vi "Get Calibration Info.vi"(4 "출장교정 List":refnum<vi>, 5 "교정환경 in":T1, 6 "교정절차 목록 List":refnum<vi>, 7 "교정정보 in":T2 caption="입력 클러스터", 8 "에러 입력(에러 없음)":errorcluster, 9 "콤보박스 참조":refnum<vi>[](array[refnum]), 10 "현장리스트?":bool, 11 "등록번호":string) -> (0 "에러 출력":errorcluster, 1 "교정환경 out":T1, 2 "교정정보 out":T2 caption="출력 클러스터", 3 "기타정보":string[](array[string]))   [LabVIEW 2020]
uses:
  Controls/Clst_Cal Info Global.ctl
  Controls/Clst_Atm Info Global.ctl
  <vilib>/addons/database/NI_Database_API.lvlib
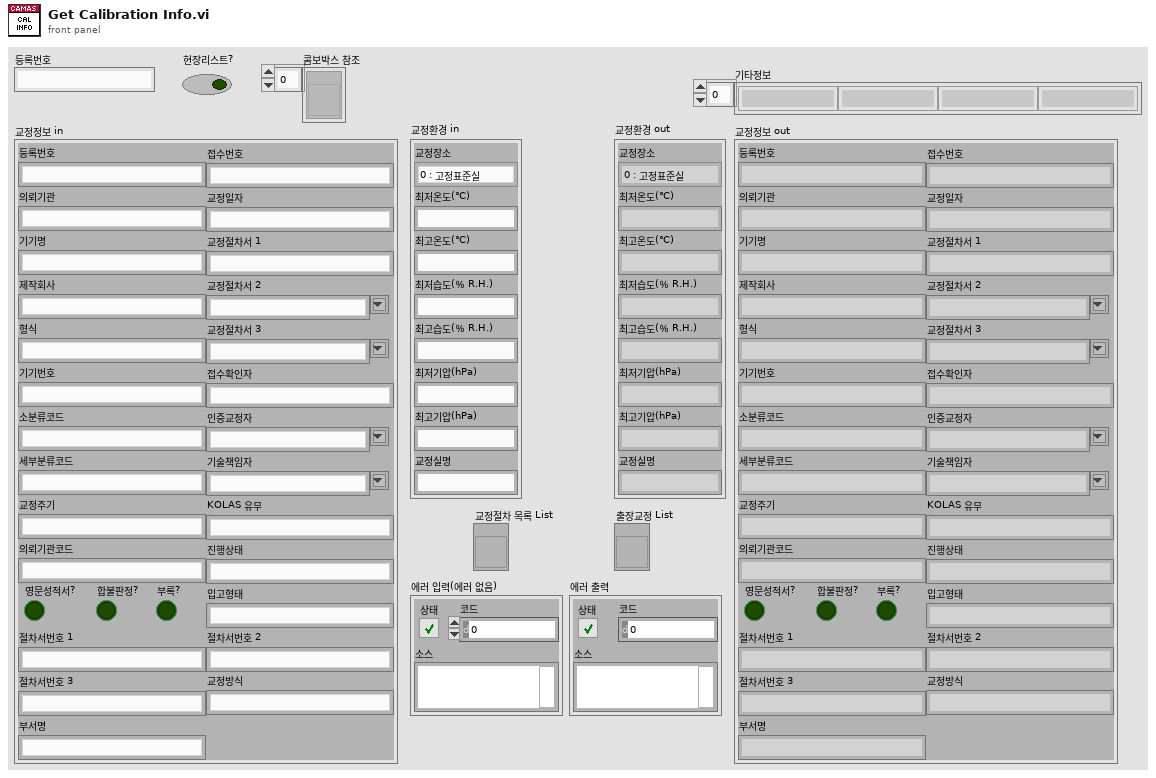
[diagram p1: front panel]
types:
  T1 = typedef "Clst_Atm Info Global.ctl" = cluster{"교정장소":enum16{"0 : 고정표준실", "1 : 현장교정"}, "최저온도(℃)":string, "최고온도(℃)":string, "최저습도(％ R.H.)":string, "최고습도(％ R.H.)":string, "최저기압(hPa)":string, "최고기압(hPa)":string, "교정실명":string}
  T2 = typedef "Clst_Cal Info Global.ctl" = cluster{"등록번호":string, "의뢰기관":string, "기기명":string, "제작회사":string, "형식":string, "기기번호":string, "소분류코드":string, "세부분류코드":string, "교정주기":string, "접수번호":string, "교정일자":string, "교정절차서 1":string, "교정절차서 2":string, "교정절차서 3":string, "접수확인자":string, "인증교정자":string, "기술책임자":string, "KOLAS 유무":string, "진행상태":string, "의뢰기관코드":string, "입고형태":string, "영문성적서?":bool, "합불판정?":bool, "부록?":bool, "절차서번호 1":string, "절차서번호 2":string, "절차서번호 3":string, "교정방식":string, "부서명":string}
  T3 = typedef "NI_Database_API.lvlib/Conn ObjectReference.ctl" = refnum<k1>
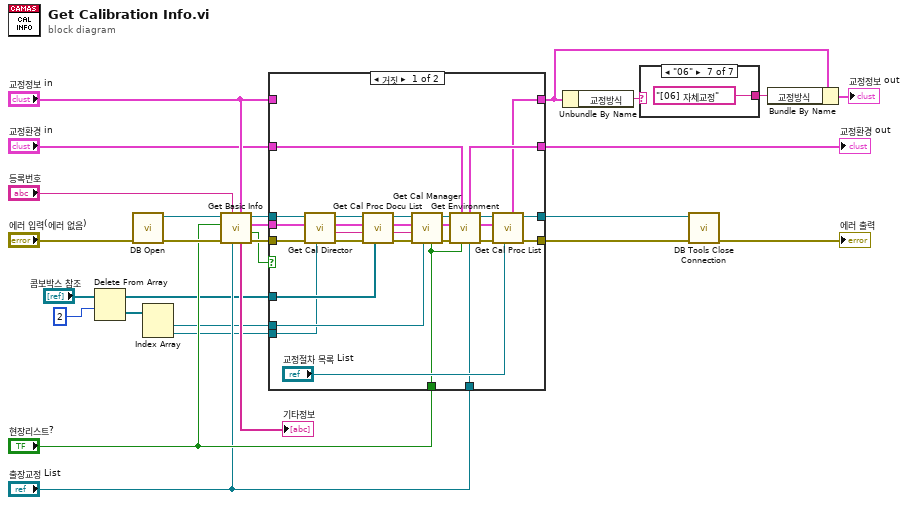
[diagram p0: block diagram]
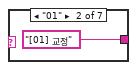
[diagram p3: hidden frame]
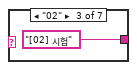
[diagram p4: hidden frame]
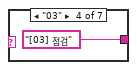
[diagram p5: hidden frame]
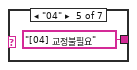
[diagram p6: hidden frame]
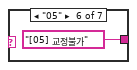
[diagram p7: hidden frame]
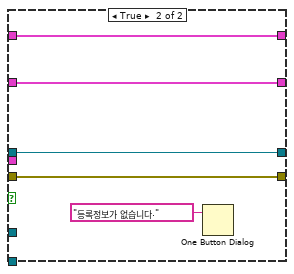
[diagram p8: hidden frame]
diagram:
  n1 = Delete From Array(array="콤보박스 참조", length=2 ("길이")) -> (deleted portion=w9:refnum<vi>[], array with subset deleted=w7:refnum<vi>[])  [unwired: 1 in]
  n2 = call "DB Open.vi"("에러 입력"="에러 입력(에러 없음)") -> ("에러 출력"=w26:errorcluster, "참조 번호 출력"=w27:T3)  [unwired: 9 in]
  n3 = Index Array(array=w9) -> (element #1=w6:refnum<vi>, element #2=w5:refnum<vi>)  [unwired: 2 in]
  n4 = call "Get Basic Info.vi"("교정정보 in"="교정정보 in", "출장교정 List"="출장교정 List", "등록번호"="등록번호", "에러 입력(에러 없음)"=w26, "현장리스트?"="현장리스트?", "참조 번호 입력"=w27) -> ("에러 출력"=w24:errorcluster, "None?"=w20:bool, "교정정보 out"=w22:T2, "참조 번호 출력"=w23:T3, "기타정보"=→"기타정보":string[])  [unwired: 1 in]
  n5 = case shown="거짓" w20 {
    tunnel: w24 -> [w55 w60]
    tunnel: w23 -> [w53 w59]
    tunnel: w22 -> [w51 _]
    tunnel: [w40 w59] -> w16
    tunnel: [w42 w60] -> w15
    tunnel: [w37 w57] -> w3
    tunnel: "교정정보 in" -> [_ w57]
    tunnel: [w39 w56] -> w18
    tunnel: "교정환경 in" -> [w44 w56]
    tunnel: "현장리스트?" -> [w34 _]
    tunnel: "출장교정 List" -> [w35 _]
    tunnel: w7 -> [w33 _]
    tunnel: w6 -> [w32 _]
    tunnel: w5 -> [w31 _]
    frame False {
      n6 = call "Get Cal Director.vi"("기술책임자 참조"=w31, "에러 입력(에러 없음)"=w55, "교정정보 in"=w51, "참조 번호 입력"=w53) -> ("에러 출력"=w54:errorcluster, "기책 사번"=w50:string, "교정정보 out"=w29:T2, "참조 번호 출력"=w52:T3)  [unwired: 4 in]
      n7 = call "Get Cal Proc Docu List.vi"("교정절차서 참조 배열"=w33, "에러 입력(에러 없음)"=w54, "기책 사번"=w50, "교정정보 in"=w29, "참조 번호 입력"=w52) -> ("에러 출력"=w49:errorcluster, "기책 사번 out"=w30:string, "교정정보 out"=w28:T2, "참조 번호 출력"=w48:T3)  [unwired: 3 in]
      n8 = call "Get Cal Manager.vi"("현장리스트?"=w34, "인증교정자 참조"=w32, "에러 입력(에러 없음)"=w49, "기책사번"=w30, "교정정보 in"=w28, "참조 번호 입력"=w48) -> ("에러 출력"=w47:errorcluster, "교정정보 out"=w45:T2, "참조 번호 출력"=w46:T3)  [unwired: 3 in]
      n9 = call "Get Environment.vi"("출장교정 List"=w35, "현장리스트?"=w34, "교정환경 in"=w44, "에러 입력(에러 없음)"=w47, "교정정보 in"=w45, "참조 번호 입력"=w46) -> ("에러 출력"=w43:errorcluster, "교정정보 out"=w38:T2, "참조 번호 출력"=w41:T3, "교정환경out"=w39:T1)  [unwired: 2 in]
      n10 = call "Get Cal Proc List.vi"("교정절차 목록 MC List"="교정절차 목록 List", "에러 입력(에러 없음)"=w43, "교정정보 in"=w38, "참조 번호 입력"=w41) -> ("에러 출력"=w42:errorcluster, "참조 번호 출력"=w40:T3, "교정정보 out"=w37:T2)  [unwired: 5 in]
    }
    frame True {
      n11 = One Button Dialog(message="등록정보가 없습니다." ("메시지")) -> ()  [unwired: 1 in, 1 out]
    }
  }
  "교정환경 out" <- w18
  n12 = Unbundle By Name(w3) -> ("교정방식"=w4:string)
  n13 = case shown="\"06\"" w4 {
    tunnel: [_ "[01] 교정" "[02] 시험" "[03] 점검" "[04] 교정불필요" "[05] 교정불가" "[06] 자체교정"] -> w2
    frame Default {
    }
    frame "01" {
    }
    frame "02" {
    }
    frame "03" {
    }
    frame "04" {
    }
    frame "05" {
    }
    frame "06" {
    }
  }
  n14 = call <vilib>:"DB Tools Close Connection.vi"("error in (no error)"=w15, "connection reference"=w16) -> ("error out"=→"에러 출력":errorcluster)  [unwired: 5 in]
  n15 = Bundle By Name(cluster=w3, "교정방식"=w2) -> (→"교정정보 out":T2)
